vi "LWXPS_ReferencingActionListGet.vi"(0 "XPS Reference IN":refnum<k24>, 11 "LabVIEW error IN":errorcluster) -> (4 "XPS Reference OUT":refnum<k24>, 6 "Returned error code":i32, 8 "List":string, 10 "XPS Error String":string, 15 "LabVIEW error OUT":errorcluster)   [LabVIEW 2014]
uses:
  D:/XPSQ8_LabView_Library/Development/Source/Dll/Newport.XPS.CommandInterface.dll
  Dll/Newport.XPS.CommandInterface.dll
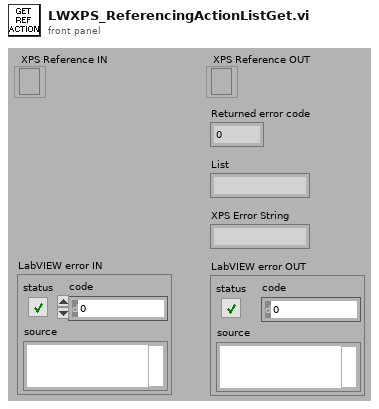
[diagram p1: front panel]
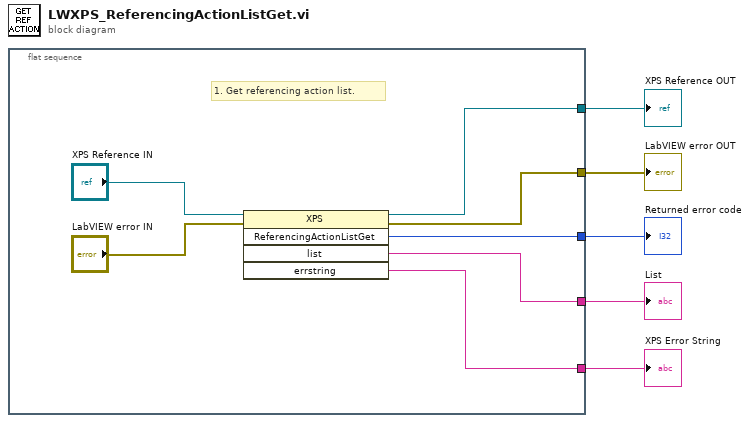
[diagram p0: block diagram]
diagram:
  n1 = flat-sequence {
    tunnel: [w10] -> w5
    tunnel: [w8] -> w4
    tunnel: [w11] -> w3
    tunnel: [w7] -> w2
    tunnel: [w6] -> w1
    frame #0 {
      # "1. Get referencing action list."
      n2 = invoke class="XPS" method="ReferencingActionListGet"(reference="XPS Reference IN", error in="LabVIEW error IN") -> (reference out=w10:refnum<k24>, error out=w8:errorcluster, "ReferencingActionListGet"=w11:i32, "list"=w6:string, "errstring"=w7:string)  [unwired: 3 in]
    }
  }
  "XPS Error String" <- w2
  "XPS Reference OUT" <- w5
  "LabVIEW error OUT" <- w4
  "Returned error code" <- w3
  "List" <- w1
